vi "PIM Unflatten Test Parameters.vi"(9 "error in (no error)":errorcluster, 10 "Parameter String":string) -> (1 "error out":errorcluster, 2 "PIM Test Parameters":T2={"Stimulus"={"C1 Pwr dBm"=0.0, "C2 Pwr dBm"=0.0, "Power Units"=enum."dBm", "Meas Type"=enum."Time", "C1 Freq MHz"=0.0, "C2 Freq MHz"=0.0, "Swept Freq Step"=0}, "Measure"={"IM Order"=0, "Direction"=0, "Averaging"=1, "ALC ON?"=TRUE, "Peak Hold?"=TRUE, "Peak last N"=1, "Ref Level dBm"=-100.0, "Ref Units"=enum."dBm", "Num Samples"=1, "Sample units"=enum."Sample(s)", "Update Rate (s)"=0.0, "DUT PORT"=enum."Port 1", "Percent (%)"=100}, "Display"={"Power Scale"={"yRange_min"=0, "yRange_max"=0}, "xRange_span"=5}} {"Stimulus"."Swept Freq Step" items=[".2", ".4", "1.0", "2.0"]; "Measure"."Averaging" items=["None", "Minimum", "Normal", "High", "Maximum"]; "Measure"."Direction" items=["Reverse", "Forward", "Auxiliary"]; "Measure"."IM Order" items=["3rd", "5th", "7th", "9th", "11th", "13th", "15th", "17th", "19th", "21st", "23rd", "25th", "27th", "29th", "31st", "33rd"]}, 5 "Test Version":string)   [LabVIEW 2011]
uses:
  TypeDefs/PIM Test Parameters.ctl
  TypeDefs/PIM Stimulus Parameters.ctl
  BPIMCore/HW IO/PIM Sweep Step Size.ctl
  TypeDefs/PIM Measurement Parameters.ctl
  BPIMCore/HW IO/IMOrder.ctl
  BPIMCore/HW IO/MeasMode.ctl
  BPIMCore/HW IO/HW Averaging.ctl
  TypeDefs/PIM Meas Units.ctl
  BPIMCore/HW IO/DUTport.ctl
  TypeDefs/PIM Display Parameters.ctl
  Test Return Parameter.ctl
  TypeDefs/PIM Test Parameters v1.0.ctl
  TypeDefs/PIM Test Parameters v1.1.ctl
  TypeDefs/PIM Test Parameters v1.2-1.3.ctl
  TypeDefs/PIM Test Parameters v2.0-6.1.ctl
panel:
  in  "Return Parameter":T1
  out "Parameter Variant":variant
  in  "Required Instruments":string[](array[string])=["PIM"]
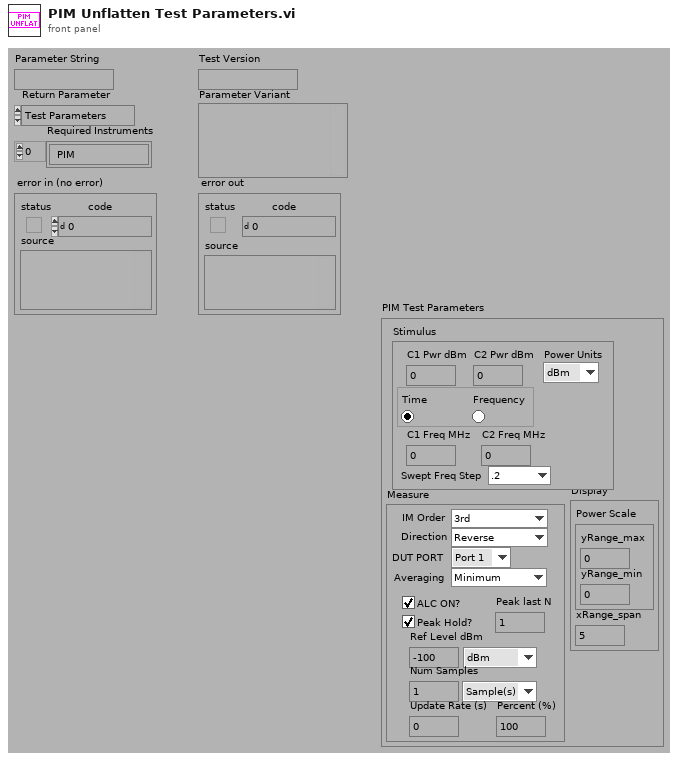
[diagram p1: front panel]
types:
  T1 = typedef "Test Return Parameter.ctl" = enum16{"Test Parameters", "Required Instruments", "Datasheets", "QuickMode"}
  T2 = typedef "PIM Test Parameters.ctl" = cluster{"Stimulus":T3, "Measure":T5, "Display":T11}
  T3 = typedef "PIM Stimulus Parameters.ctl" = cluster{"C1 Pwr dBm":dbl, "C2 Pwr dBm":dbl, "Power Units":enum16{"dBm", "Watts"}, "Meas Type":enum32{"Time", "Frequency"}, "C1 Freq MHz":dbl, "C2 Freq MHz":dbl, "Swept Freq Step":T4}
  T4 = typedef "PIM Sweep Step Size.ctl" = u16
  T5 = typedef "PIM Measurement Parameters.ctl" = cluster{"IM Order":T6, "Direction":T7, "Averaging":T8, "ALC ON?":bool, "Peak Hold?":bool, "Peak last N":u32, "Ref Level dBm":dbl, "Ref Units":enum16{"dBm", "dBc"}, "Num Samples":u32, "Sample units":T9, "Update Rate (s)":dbl, "DUT PORT":T10, "Percent (%)":u8}
  T6 = typedef "IMOrder.ctl" = u8
  T7 = typedef "MeasMode.ctl" = u16
  T8 = typedef "HW Averaging.ctl" = u16
  T9 = typedef "PIM Meas Units.ctl" = enum16{"Sample(s)", "Second(s)", "Sweep(s)"}
  T10 = typedef "DUTport.ctl" = enum16{"Port 1", "Port 2"}
  T11 = typedef "PIM Display Parameters.ctl" = cluster{"Power Scale":cluster{"yRange_min":i32, "yRange_max":i32}, "xRange_span":u32}
  T12 = typedef "PIM Test Parameters v1.0.ctl" = cluster{"Step Tag":string, "Quickmode?":bool, "PIM Test Stimulus":cluster{"C1 Pwr dBm":dbl, "C2 Pwr dBm":dbl, "Power Units":enum16{"dBm", "Watts"}, "Meas Type":enum32{"Band Edges", "Fixed Pair", "Swept Freq"}, "C1 Fixed MHz":dbl, "C2 Fixed MHz":dbl, "Swept Freq Step":u16}, "Measure":cluster{"IM Order":u8, "Direction":u16, "Averaging":u16, "ALC ON?":bool, "Peak Hold?":bool, "Peak last N":u32, "Ref Level dBm":dbl, "Ref Units":enum16{"dBm", "dBc"}, "Num Samples":u32, "Sample units":enum16{"Sample(s)", "Second(s)", "Sweep(s)"}, "Update Rate (s)":dbl}, "Display":cluster{"Power Scale":cluster{"yRange_min":i32, "yRange_max":i32}, "xRange_span":u32}, "Datasheets":cluster{"Datasheets to Generate":i32[], "Print Datasheets":bool}}
  T13 = typedef "PIM Test Parameters v1.1.ctl" = cluster{"PIM Test Stimulus":cluster{"C1 Pwr dBm":dbl, "C2 Pwr dBm":dbl, "Power Units":enum16{"dBm", "Watts"}, "Meas Type":enum32{"Band Edges", "Fixed Pair", "Swept Freq"}, "C1 Fixed MHz":dbl, "C2 Fixed MHz":dbl, "Swept Freq Step":u16}, "Measure":cluster{"IM Order":u8, "Direction":u16, "Averaging":u16, "ALC ON?":bool, "Peak Hold?":bool, "Peak last N":u32, "Ref Level dBm":dbl, "Ref Units":enum16{"dBm", "dBc"}, "Num Samples":u32, "Sample units":enum16{"Sample(s)", "Second(s)", "Sweep(s)"}, "Update Rate (s)":dbl}, "Display":cluster{"Power Scale":cluster{"yRange_min":i32, "yRange_max":i32}, "xRange_span":u32}, "Datasheets":cluster{"Datasheet to Generate":i32, "Print Datasheets":bool}[]}
  T14 = typedef "PIM Test Parameters v1.2-1.3.ctl" = cluster{"Stimulus":cluster{"C1 Pwr dBm":dbl, "C2 Pwr dBm":dbl, "Power Units":enum16{"dBm", "Watts"}, "Meas Type":enum32{"Band Edges", "Fixed Pair", "Swept Freq"}, "C1 Fixed MHz":dbl, "C2 Fixed MHz":dbl, "Swept Freq Step":u16}, "Measure":cluster{"IM Order":T6, "Direction":T7, "Averaging":T8, "ALC ON?":bool, "Peak Hold?":bool, "Peak last N":u32, "Ref Level dBm":dbl, "Ref Units":enum16{"dBm", "dBc"}, "Num Samples":u32, "Sample units":T9, "Update Rate (s)":dbl}, "Display":T11}
  T15 = typedef "PIM Test Parameters v2.0-6.1.ctl" = cluster{"Stimulus":cluster{"C1 Pwr dBm":dbl, "C2 Pwr dBm":dbl, "Power Units":enum16{"dBm", "Watts"}, "Meas Type":enum32{"Time", "Frequency"}, "C1 Freq MHz":dbl, "C2 Freq MHz":dbl, "Swept Freq Step":u16}, "Measure":cluster{"IM Order":u8, "Direction":u16, "Averaging":u16, "ALC ON?":bool, "Peak Hold?":bool, "Peak last N":u32, "Ref Level dBm":dbl, "Ref Units":enum16{"dBm", "dBc"}, "Num Samples":u32, "Sample units":enum16{"Sample(s)", "Second(s)", "Sweep(s)"}, "Update Rate (s)":dbl, "DUT PORT":enum16{"Port 1", "Port 2"}}, "Display":cluster{"Power Scale":cluster{"yRange_min":i32, "yRange_max":i32}, "xRange_span":u32}}
  T16 = typedef "Test Datasheets v1.0-4.0.ctl" = cluster{"Datasheet to Generate":i32, "Print Datasheets":bool}[]
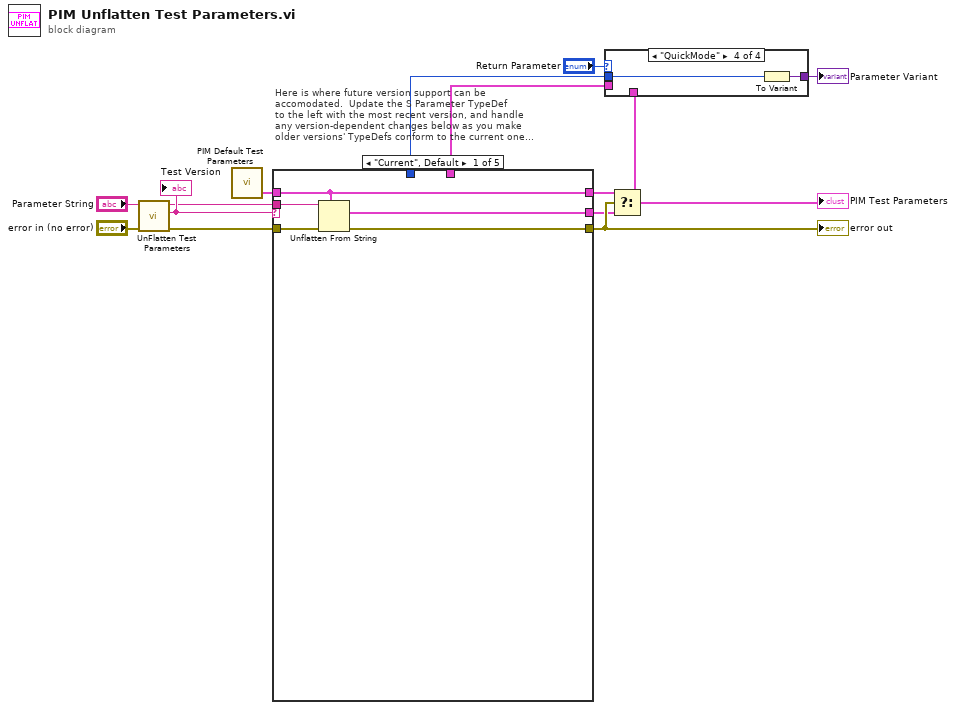
[diagram p0: block diagram]
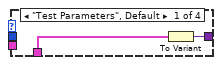
[diagram p2: hidden frame]
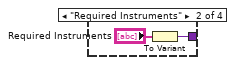
[diagram p3: hidden frame]
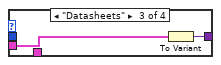
[diagram p4: hidden frame]
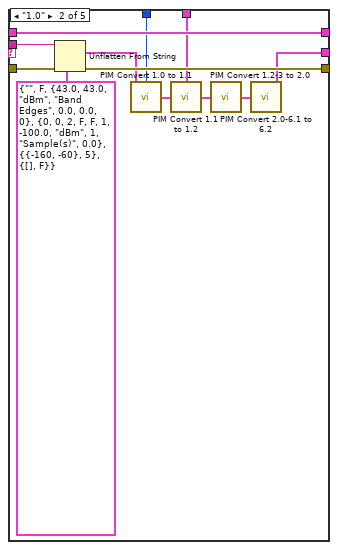
[diagram p5: hidden frame]
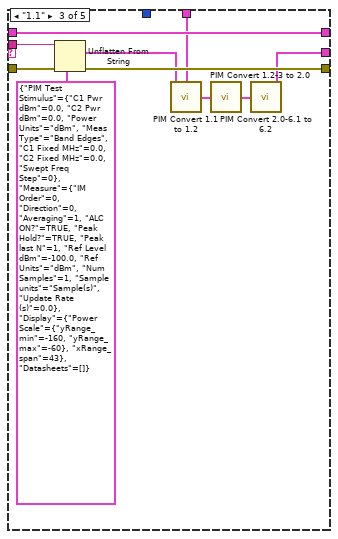
[diagram p6: hidden frame]
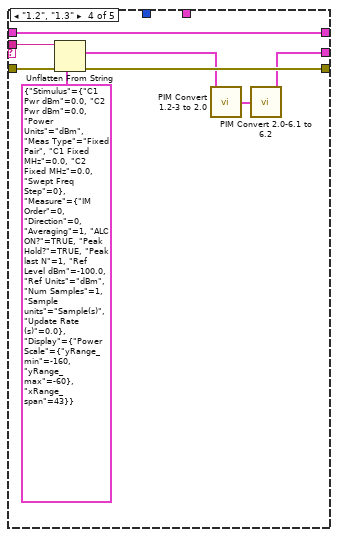
[diagram p7: hidden frame]
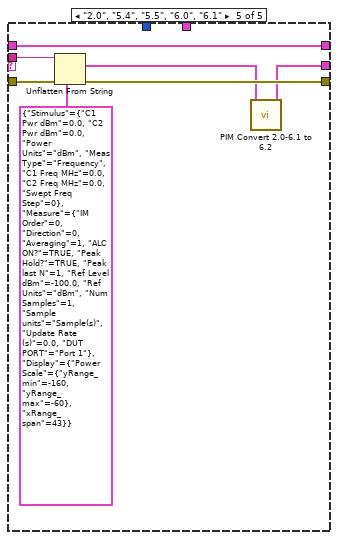
[diagram p8: hidden frame]
diagram:
  # "Here is where future version support can be\naccomodated.  Update the S Parameter TypeDef\nto the left with the most recent version, and handle\nany version-dependent changes below as you make\nolder versions' TypeDefs conform to the current one..."
  n1 = call "UnFlatten Test Parameters.vi"("error in (no error)"="error in (no error)", "Flattened Test Parameters with Version (\"\")"="Parameter String") -> ("error out"=w5:errorcluster, "Test Version"=w13:string, "Flat Test Parameters"=w12:string)  [unwired: 3 out]
  "Test Version" <- w13
  n2 = call "PIM Default Test Parameters.vi"() -> ("Default PIM Test Parameters"=w1:T2)
  n3 = case shown="\"Current\", Default" w13 {
    tunnel: w12 -> [w19 w31 w41 w49 w56]
    tunnel: w1 -> [w16 w29 w39 w47 w54]
    tunnel: [w18 w30 w40 w48 w55] -> w8
    tunnel: [w16 w29 w39 w47 w54] -> w11
    tunnel: w5 -> [w15 w28 w38 w46 w53]
    tunnel: [_ w25 _ _ _] -> w4
    tunnel: [_ w24 w36 _ _] -> w3
    tunnel: [w17 w20 w32 w42 w50] -> w2
    frame "Current", Default {
      n4 = Unflatten From String(type=w16, binary string=w19, error in (no error)=w15) -> (value=w17:T2, error out=w18:errorcluster)  [unwired: 3 out]
    }
    frame "1.0" {
      n5 = Unflatten From String(type=T12 {"Step Tag"="", "Quickmode?"=FALSE, "PIM Test Stimulus"={"C1 Pwr dBm"=43.0, "C2 Pwr dBm"=43.0, "Power Units"=enum."dBm", "Meas Type"=enum."Band Edges", "C1 Fixed MHz"=0.0, "C2 Fixed MHz"=0.0, "Swept Freq Step"=0}, "Measure"={"IM Order"=0, "Direction"=0, "Averaging"=2, "ALC ON?"=FALSE, "Peak Hold?"=FALSE, "Peak last N"=1, "Ref Level dBm"=-100.0, "Ref Units"=enum."dBm", "Num Samples"=1, "Sample units"=enum."Sample(s)", "Update Rate (s)"=0.0}, "Display"={"Power Scale"={"yRange_min"=-160, "yRange_max"=-60}, "xRange_span"=5}, "Datasheets"={"Datasheets to Generate"=[], "Print Datasheets"=FALSE}} ("PIM Test Parameters"), binary string=w31, error in (no error)=w28) -> (value=w26:T12, error out=w30:errorcluster)  [unwired: 3 out]
      n6 = call "PIM Convert 1.0 to 1.1.vi"("PIM 1.0 Test Parameters"=w26) -> ("QuickMode"=w25:i8, "PIM 1.1 Test Parameters"=w23:T13)
      n7 = call "PIM Convert 1.1 to 1.2.vi"("PIM 1.1 Test Parameters"=w23) -> ("Datasheets"=w24:T16, "PIM 1.2 Test Parameters"=w22:T14)
      n8 = call "PIM Convert 1.2-3 to 2.0.vi"("PIM 1.2/3 Test Parameters"=w22) -> ("PIM 2.0 Test Parameters"=w21:T15)  [unwired: 1 out]
      n9 = call "PIM Convert 2.0-6.1 to 6.2.vi"("PIM 2.0 - 6.1 Test Parameters"=w21) -> ("PIM Test Parameters"=w20:T2)  [unwired: 1 in]
    }
    frame "1.1" {
      n10 = Unflatten From String(type=T13 {"PIM Test Stimulus"={"C1 Pwr dBm"=0.0, "C2 Pwr dBm"=0.0, "Power Units"=enum."dBm", "Meas Type"=enum."Band Edges", "C1 Fixed MHz"=0.0, "C2 Fixed MHz"=0.0, "Swept Freq Step"=0}, "Measure"={"IM Order"=0, "Direction"=0, "Averaging"=1, "ALC ON?"=TRUE, "Peak Hold?"=TRUE, "Peak last N"=1, "Ref Level dBm"=-100.0, "Ref Units"=enum."dBm", "Num Samples"=1, "Sample units"=enum."Sample(s)", "Update Rate (s)"=0.0}, "Display"={"Power Scale"={"yRange_min"=-160, "yRange_max"=-60}, "xRange_span"=43}, "Datasheets"=[]} ("PIM Test Parameters"), binary string=w41, error in (no error)=w38) -> (value=w35:T13, error out=w40:errorcluster)  [unwired: 3 out]
      n11 = call "PIM Convert 1.1 to 1.2.vi"("PIM 1.1 Test Parameters"=w35) -> ("Datasheets"=w36:T16, "PIM 1.2 Test Parameters"=w34:T14)
      n12 = call "PIM Convert 1.2-3 to 2.0.vi"("PIM 1.2/3 Test Parameters"=w34) -> ("PIM 2.0 Test Parameters"=w33:T15)  [unwired: 1 out]
      n13 = call "PIM Convert 2.0-6.1 to 6.2.vi"("PIM 2.0 - 6.1 Test Parameters"=w33) -> ("PIM Test Parameters"=w32:T2)  [unwired: 1 in]
    }
    frame "1.2", "1.3" {
      n14 = Unflatten From String(type=T14 {"Stimulus"={"C1 Pwr dBm"=0.0, "C2 Pwr dBm"=0.0, "Power Units"=enum."dBm", "Meas Type"=enum."Fixed Pair", "C1 Fixed MHz"=0.0, "C2 Fixed MHz"=0.0, "Swept Freq Step"=0}, "Measure"={"IM Order"=0, "Direction"=0, "Averaging"=1, "ALC ON?"=TRUE, "Peak Hold?"=TRUE, "Peak last N"=1, "Ref Level dBm"=-100.0, "Ref Units"=enum."dBm", "Num Samples"=1, "Sample units"=enum."Sample(s)", "Update Rate (s)"=0.0}, "Display"={"Power Scale"={"yRange_min"=-160, "yRange_max"=-60}, "xRange_span"=43}} ("PIM 1.2 Test Parameters"), binary string=w49, error in (no error)=w46) -> (value=w44:T14, error out=w48:errorcluster)  [unwired: 3 out]
      n15 = call "PIM Convert 1.2-3 to 2.0.vi"("PIM 1.2/3 Test Parameters"=w44) -> ("PIM 2.0 Test Parameters"=w43:T15)  [unwired: 1 out]
      n16 = call "PIM Convert 2.0-6.1 to 6.2.vi"("PIM 2.0 - 6.1 Test Parameters"=w43) -> ("PIM Test Parameters"=w42:T2)  [unwired: 1 in]
    }
    frame "2.0", "5.4", "5.5", "6.0", "6.1" {
      n17 = Unflatten From String(type=T15 {"Stimulus"={"C1 Pwr dBm"=0.0, "C2 Pwr dBm"=0.0, "Power Units"=enum."dBm", "Meas Type"=enum."Frequency", "C1 Freq MHz"=0.0, "C2 Freq MHz"=0.0, "Swept Freq Step"=0}, "Measure"={"IM Order"=0, "Direction"=0, "Averaging"=1, "ALC ON?"=TRUE, "Peak Hold?"=TRUE, "Peak last N"=1, "Ref Level dBm"=-100.0, "Ref Units"=enum."dBm", "Num Samples"=1, "Sample units"=enum."Sample(s)", "Update Rate (s)"=0.0, "DUT PORT"=enum."Port 1"}, "Display"={"Power Scale"={"yRange_min"=-160, "yRange_max"=-60}, "xRange_span"=43}} ("PIM Test Parameters"), binary string=w56, error in (no error)=w53) -> (value=w51:T15, error out=w55:errorcluster)  [unwired: 3 out]
      n18 = call "PIM Convert 2.0-6.1 to 6.2.vi"("PIM 2.0 - 6.1 Test Parameters"=w51) -> ("PIM Test Parameters"=w50:T2)  [unwired: 1 in]
    }
  }
  "error out" <- w8
  n19 = Select(t=w11, s=w8, f=w2) -> (s? t:f=w7:T2)
  "PIM Test Parameters" <- w7
  n20 = case shown="\"QuickMode\"" "Return Parameter" {
    tunnel: [w58 w60 w62 w64] -> w9
    tunnel: w7 -> [w57 _ _ _]
    tunnel: w4 -> [_ _ _ w63]
    tunnel: w3 -> [_ _ w61 _]
    frame "Test Parameters", Default {
      n21 = To Variant(anything=w57) -> (Variant=w58:variant)
    }
    frame "Required Instruments" {
      n22 = To Variant(anything="Required Instruments") -> (Variant=w60:variant)
    }
    frame "Datasheets" {
      n23 = To Variant(anything=w61) -> (Variant=w62:variant)
    }
    frame "QuickMode" {
      n24 = To Variant(anything=w63) -> (Variant=w64:variant)
    }
  }
  "Parameter Variant" <- w9
